vi "Open_File.vi"(8 "error in (no error)":errorcluster, 11 "Logger_Data In":T1) -> (0 "error out":errorcluster, 3 "Logger_Data Out":T1)   [LabVIEW 2019, in "Data_Logger.lvlib"]
uses:
  Data_Logger.lvlib
  Logger_Data.ctl
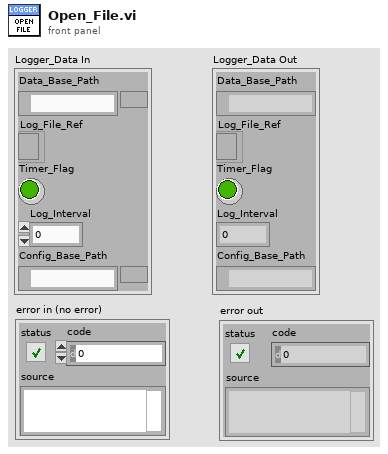
[diagram p1: front panel]
types:
  T1 = typedef "Data_Logger.lvlib/Logger_Data.ctl" = cluster{"Data_Base_Path":path, "Log_File_Ref":refnum<file>, "Timer_Flag":bool, "Log_Interval":dbl, "Config_Base_Path":path}
  T2 = enum16{"open", "replace", "create", "open or create", "replace or create", "replace or create with confirmation"}
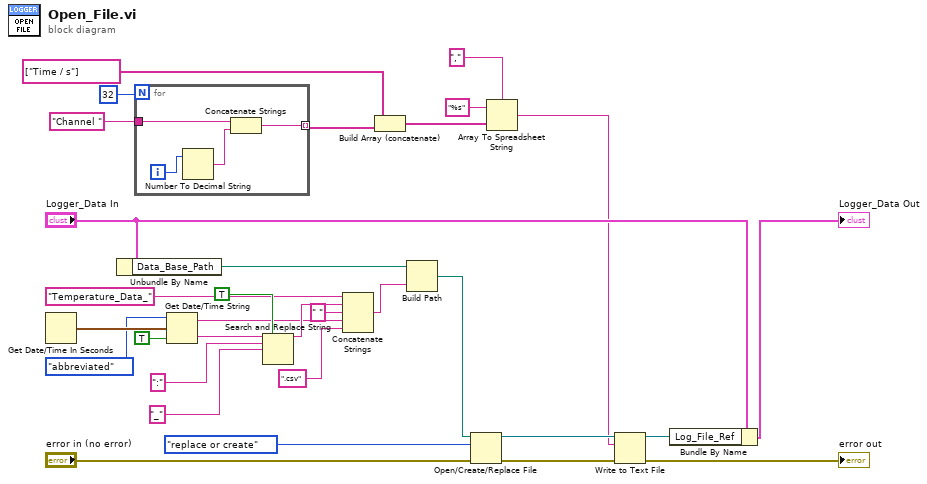
[diagram p0: block diagram]
diagram:
  n1 = Get Date/Time In Seconds() -> (seconds since 1Jan1904=w28:timestamp)
  n2 = Unbundle By Name("Logger_Data In") -> ("Data_Base_Path"=w29:path)
  n3 = for {
    N: 32 -> [_]
    tunnel: "Channel " -> [w35]
    tunnel: [w32] -> w8 mode=indexing
    i -> [w34]
    n4 = Number To Decimal String(number=w34) -> (decimal integer string=w33:string)  [unwired: 1 in]
    n5 = Concatenate Strings(w35, w33) -> (w32:string)
  }
  n6 = Get Date/Time String(date format (0)=enum16{"short", "long", "abbreviated"}."abbreviated", seconds (now)=w28, want seconds? (F)=TRUE) -> (date string=w17:string, time string=w25:string)
  n7 = Search and Replace String(replace all?=TRUE ("replace all? (F)"), input string=w25, search string=":", replace string="_" ("replace string (\"\")")) -> (result string=w21:string)  [unwired: 4 in, 3 out]
  n8 = Concatenate Strings("Temperature_Data_" ("string"), w21, " " ("string"), w17, ".csv" ("string")) -> (w20:string)
  n9 = Build Array (concatenate)(string[] ["Time / s"] ("array"), w8) -> (w6:string[])
  n10 = Build Path(base path=w29, name or relative path=w20) -> (appended path=w30:path)
  n11 = Open/Create/Replace File(file path (use dialog)=w30, error in="error in (no error)", operation (0:open)=T2."replace or create") -> (refnum out=w13:refnum<file>, error out=w11:errorcluster)  [unwired: 3 in, 1 out]
  n12 = Array To Spreadsheet String(delimiter (Tab)=",", array=w6, 3:"%s" ("format string")) -> (spreadsheet string=w4:string)
  n13 = Write to Text File(file (use dialog)=w13, text=w4, error in=w11) -> (refnum out=w12:refnum<file>, error out=→"error out":errorcluster)  [unwired: 1 in, 1 out]
  n14 = Bundle By Name(cluster="Logger_Data In", "Log_File_Ref"=w12) -> (→"Logger_Data Out":T1)
